vi "bats.parser.test.AddOrderLong.add.four.orders.vi"(10 "Expected OrderBook.Command[]":T2[](array[typedef])=[{"type"=enum."AddOrder", "side"=66, "orderId "=3544385890602799695, "quantity"=20000, "symbol"=4702127773838221344, "price"=9050, "executed.qty"=0, "canceled.qty"=0, "remaining.qty"=0, "seconds"=0, "nanoseconds"=447000, "Add"=FALSE, "Edit"=FALSE, "Remove"=FALSE, "seq no"=1}, {"type"=enum."AddOrder", "side"=66, "orderId "=3616443484640727631, "quantity"=200, "symbol"=4702127773838221344, "price"=9050, "executed.qty"=0, "canceled.qty"=0, "remaining.qty"=0, "seconds"=0, "nanoseconds"=547000, "Add"=FALSE, "Edit"=FALSE, "Remove"=FALSE, "seq no"=2}, {"type"=enum."AddOrder", "side"=83, "orderId "=3688501078678655567, "quantity"=50, "symbol"=4702127773838221344, "price"=9030, "executed.qty"=0, "canceled.qty"=0, "remaining.qty"=0, "seconds"=0, "nanoseconds"=647000, "Add"=FALSE, "Edit"=FALSE, "Remove"=FALSE, "seq no"=3}, {"type"=enum."AddOrder", "side"=66, "orderId "=3760558672716583503, "quantity"=150, "symbol"=4702127773838221344, "price"=19050, "executed.qty"=0, "canceled.qty"=0, "remaining.qty"=0, "seconds"=0, "nanoseconds"=747000, "Add"=FALSE, "Edit"=FALSE, "Remove"=FALSE, "seq no"=4}] {"symbol" format="%.0x"; "orderId" format="%.0x"; "side" format="%.0x"}) -> ()   [LabVIEW 2020]
uses:
  builds/fpganow.common/orderbook.command.ctl
  builds/fpganow.common/orderbook.command.type.ctl
  pitch/AddOrder/AddOrderLong.Parameters.ctl
  builds/fpganow.common/fpganow.common.fpga.lvlib
  pitch/AddOrder/AddOrderLong.lvclass
panel:
  out "Passed":bool
  in  "AddOrderLong.Parameters 4":T1={"Time Offset"=747000, "Order Id"="ORID0004", "Quantity"=150, "Symbol"="AAPL", "Side Indicator"="B", "Price"=1.905}
  in  "AddOrderLong.Parameters 3":T1={"Time Offset"=647000, "Order Id"="ORID0003", "Quantity"=50, "Symbol"="AAPL", "Side Indicator"="S", "Price"=0.903}
  in  "AddOrderLong.Parameters 2":T1={"Time Offset"=547000, "Order Id"="ORID0002", "Quantity"=200, "Symbol"="AAPL", "Side Indicator"="B", "Price"=0.905}
  in  "AddOrderLong.Parameters":T1={"Time Offset"=447000, "Order Id"="ORID0001", "Quantity"=20000, "Symbol"="AAPL", "Side Indicator"="B", "Price"=0.905}
  out "Results":T2[](array[typedef]) {"symbol" format="%.0x"; "orderId" format="%.0x"; "side" format="%.0x"}
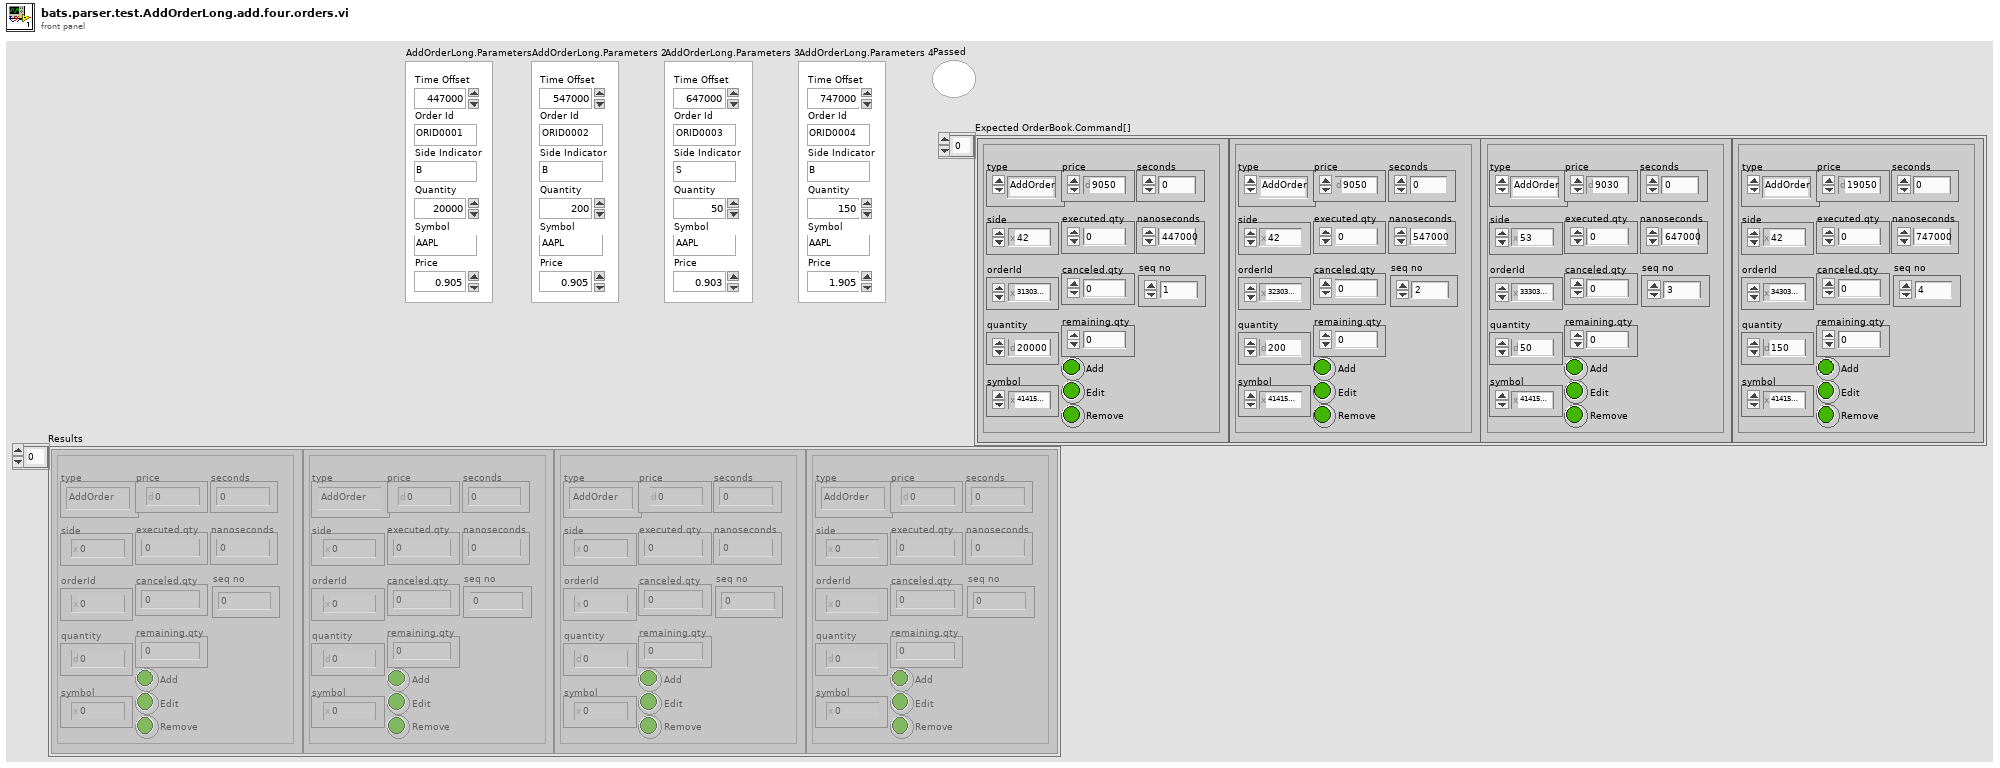
[diagram p1: front panel]
types:
  T1 = typedef "AddOrderLong.lvclass/AddOrderLong.Parameters.ctl" = cluster{"Time Offset":u32, "Order Id":string, "Quantity":u32, "Symbol":string, "Side Indicator":string, "Price":dbl}
  T2 = typedef "fpganow.common.fpga.lvlib/orderbook.command.ctl" = cluster{"type":T3, "side":u8, "orderId ":u64, "quantity":u32, "symbol":u64, "price":u64, "executed.qty":u32, "canceled.qty":u32, "remaining.qty":u32, "seconds":u64, "nanoseconds":u64, "Add":bool, "Edit":bool, "Remove":bool, "seq no":u32}
  T3 = typedef "fpganow.common.fpga.lvlib/orderbook.command.type.ctl" = enum8{"Time", "AddOrder", "OrderExecuted", "OrderExecutedAtPrice", "ReduceSize", "ModifyOrder", "DeleteOrder", "Get.Everything", "Get.All.Orders", "Get.Top"}
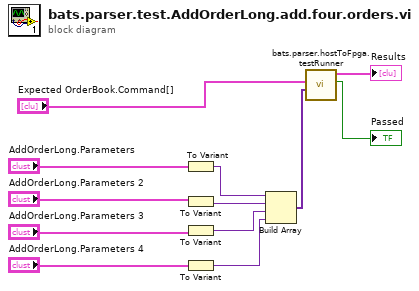
[diagram p0: block diagram]
diagram:
  n1 = To Variant(anything="AddOrderLong.Parameters") -> (Variant=w5:variant)
  n2 = To Variant(anything="AddOrderLong.Parameters 2") -> (Variant=w4:variant)
  n3 = To Variant(anything="AddOrderLong.Parameters 3") -> (Variant=w3:variant)
  n4 = To Variant(anything="AddOrderLong.Parameters 4") -> (Variant=w2:variant)
  n5 = Build Array(w5, w4, w3, w2) -> (w1:variant[])
  n6 = call "bats.parser.hostToFpga.testRunner.vi"("Test.Messages"=w1, "Expected OrderBook.Command[]"="Expected OrderBook.Command[]") -> ("Passed"=→"Passed":bool, "OrderBook.Command[]"=→"Results":T2[])  [unwired: 6 in, 2 out]
